vi "CommunicationTool.vi"(0 "VISA资源名称":refnum<visa-resource-name>="COM1", 1 "SN":string, 2 "ModelNumber":string, 5 "通信协议名称":string, 7 "Slot":T1, 9 "DelayTime":u32=1000, 11 "error in":errorcluster, 12 "Debug":bool) -> (3 "字符串数值":bool=TRUE, 4 "响应":string="ÿÿÿÿÿÿÿÿÿÿÿÿÿÿÿÿÿÿÿÿÿÿÿÿÿÿÿ", 6 "反馈结果":bool, 10 "CMD":string, 14 "data":string, 15 "error out":errorcluster)   [LabVIEW 2013]
doc: "本范例根据用户指示，对串口执行读写操作。范例运行时可按下“写入”或“读取”按钮，以及修改“读数”。\n\n设置的串口参数必须匹配连接仪器或设备的参数。本范例中，“读数”参数可指定串口读取的字节数。如端口字节超过指定的字节数，超出部分将不会被读取。如端口字节数少于指定的字节数，将返回超时错误。\n\n本范例可扩展流控制选项以包括XON和XOFF，从而允许用户选择控制字符。同时，用户可启用或禁用中止符。部分设备需要通过终止符确定命令字符串的结束位置。部分设备将发送终止符以说明待读取数据的末端。本范例演示了缓冲区中检测到终止符时，结束“读取”操作或添加终止符至“写入”数据末端的方法。"
uses:
  SystemCode/SysControl/Slot.ctl
  <vilib>/Utility/NIReport.llb/NI_report.lvclass
  SourceCode/PDINFO.ctl
  SourceCode/GlobalValue.vi
  <vilib>/Utility/error.llb/Error Cluster From Error Code.vi
  <vilib>/addons/_office/excel.llb/Excel Get Data ([str]).vi
  <vilib>/Utility/file.llb/Write To Spreadsheet File (string).vi
  <vilib>/Utility/file.llb/Read From Spreadsheet File (string).vi
  <vilib>/ErrorRing/Error Ring.xnode
  <vilib>/addons/_office/NI_ReportGenerationToolkit.lvlib
  <vilib>/Utility/NIReport.llb/Excel/NI_Excel.lvclass
panel:
  out "Time(ms)":u32
  out "SerNO":string
  out "硬件版本":string
  out "终端ID":string
  out "CCID":string="PASS"
  out "生产日期":string
  out "字符串":string
  out "x-y":u32
  out "已删除的部分":u8[](array[numeric]) format="%x"
  out "读取缓冲区":string
  out "数据Hex":string[](array[string])
  out "数据ASCII":string[](array[string])
  out "数据类型":string[](array[string])
  in  "命令列表":u16(ring)=17
  out "Write":bool
  out "Read":bool
  out "ConfigPath":string="C:\\Users\\dell\\Desktop\\ExcelReport.vi"
  out "Data":string
  out "DataType":string
  out "命令":string
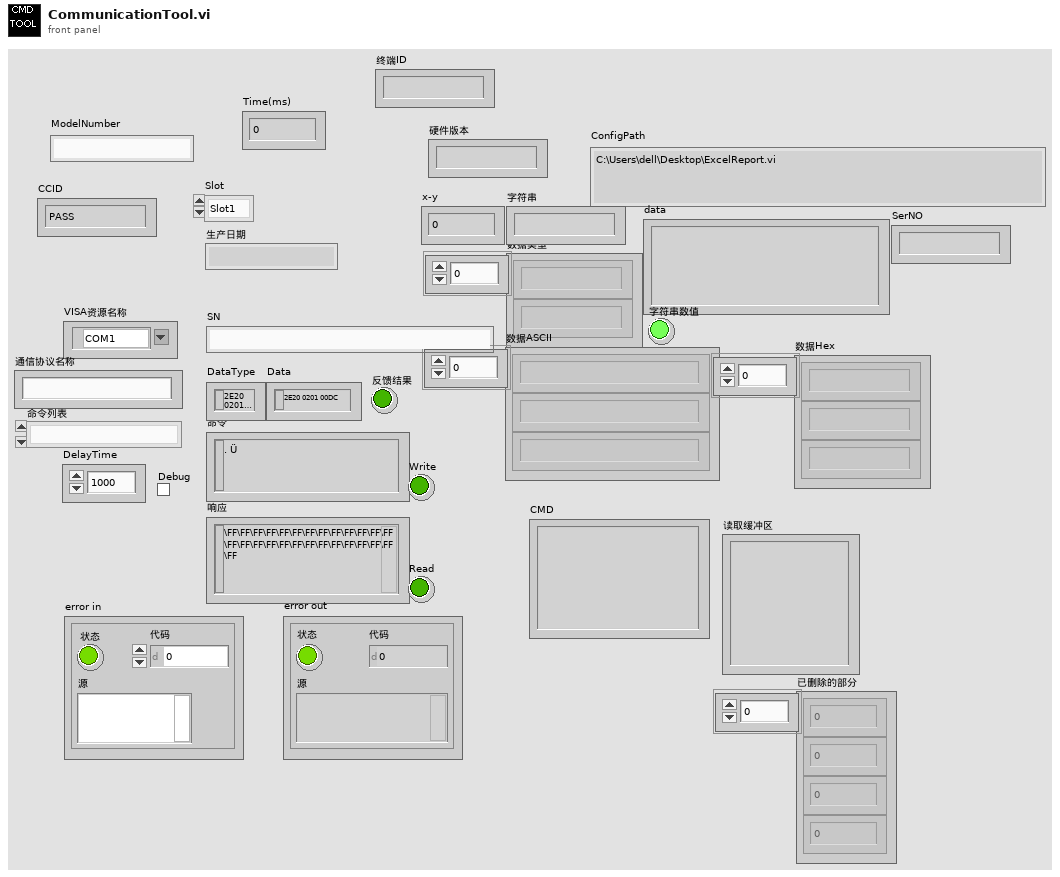
[diagram p1: front panel]
types:
  T1 = typedef "Slot.ctl" = enum16{"Slot1", "Slot2", "Slot3", "Slot4"}
  T2 = enum32{"invalid app kind", "Development System", "Run Time System", "Student Edition", "Embedded LabVIEW", "Evaluation", "Custom"}
  T3 = enum16{"maximized", "minimized", "normal", "no change"}
  T4 = enum16{"Standard Report", "HTML", "Word", "Excel"}
  T5 = typedef "PDINFO.ctl" = enum16{"Fw Ver", "HW Ver", "CCID", "WiFiName", "DevID", "SN", "TUID", "CertifID", "PdTime", "Provider", "WiFiPassword", "Imei", "AuthCode", "Reserved1", "Reserved2", "Reserved3"}
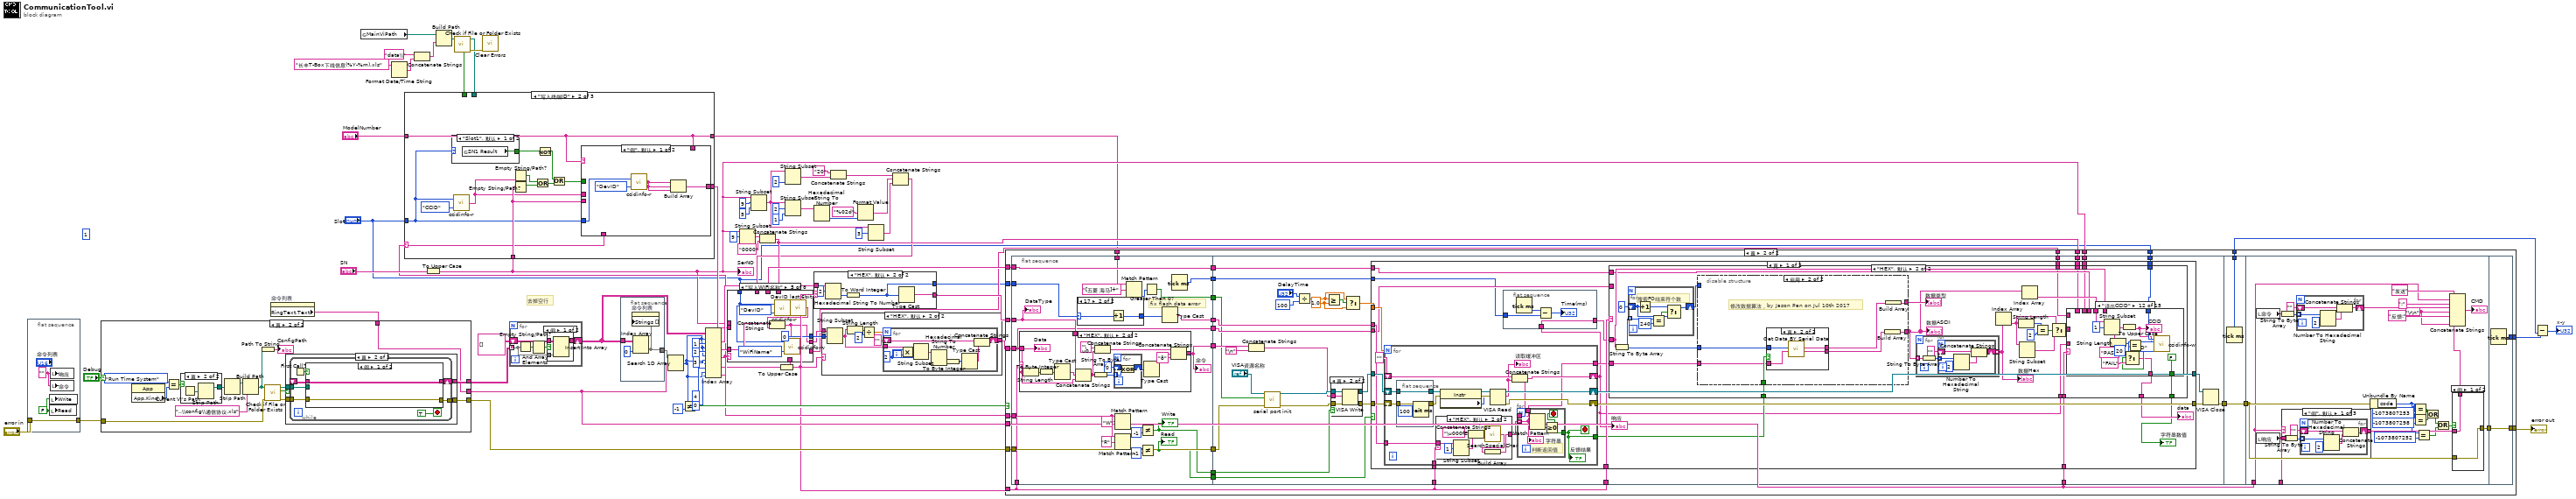
[diagram p0: block diagram]
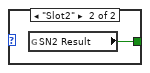
[diagram p3: hidden frame]
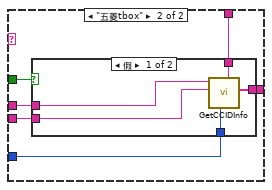
[diagram p4: hidden frame]
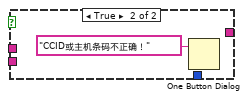
[diagram p5: hidden frame]
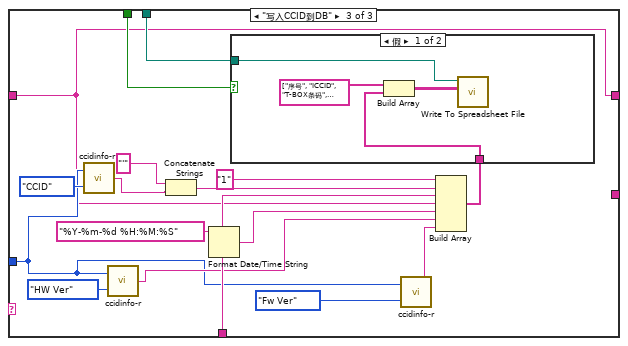
[diagram p6: hidden frame]
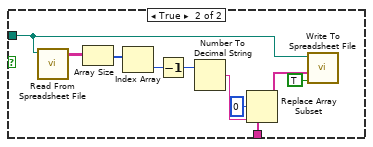
[diagram p7: hidden frame]
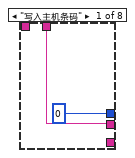
[diagram p8: hidden frame]
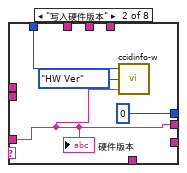
[diagram p9: hidden frame]
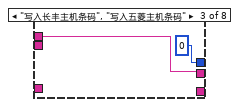
[diagram p10: hidden frame]
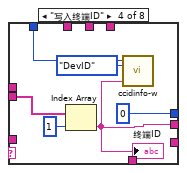
[diagram p11: hidden frame]
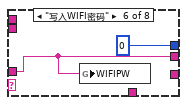
[diagram p12: hidden frame]
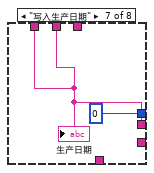
[diagram p13: hidden frame]
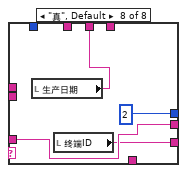
[diagram p14: hidden frame]
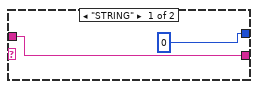
[diagram p15: hidden frame]
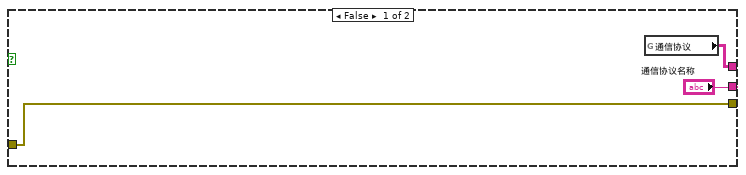
[diagram p18: hidden frame]
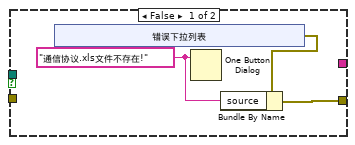
[diagram p19: hidden frame]
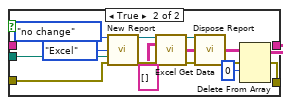
[diagram p20: hidden frame]
diagram:
  (unwired) 1
  # "去掉空行"
  n1 = flat-sequence {
    tunnel: "error in" -> [w71]
    tunnel: [w71] -> w68
    frame #0 {
      w73 = FALSE ("Read")
      w72 = "" ("响应")
      n2 = local write "Write"(w73) -> ()
      n3 = local write "Read"(w73) -> ()
      n4 = local write "响应"(w72) -> ()
      n5 = local write "命令"(w72) -> ()
    }
  }
  n6 = property on="命令列表" class="Ring (严格)"() -> ("RingText.Text"=w67:string)  [unwired: 2 in, 2 out]
  n7 = case shown="真" "Debug" {
    tunnel: [w75 w80] -> w65
    tunnel: w68 -> [w75 w79]
    tunnel: ["通信协议名称" w77] -> w56
    tunnel: [w74 w78] -> w5
    tunnel: w67 -> [_ w77]
    frame False {
      n8 = global read "GlobalValue.vi" "通信协议"() -> (w74:string[][])
    }
    frame True {
      n9 = property class="App"() -> ("App.Kind"=w89:T2)  [unwired: 2 in, 2 out]
      n10 = Equal?(x=T2."Run Time System" ("y"), y=w89) -> (x = y?=w91:bool)
      n11 = case shown="真" w91 {
        tunnel: [w125 w127] -> w90
        frame False {
          n12 = Current VI's Path() -> (path=w125:path)
        }
        frame True {
          n13 = Current VI's Path() -> (path=w126:path)
          n14 = Strip Path(path=w126) -> (stripped path=w127:path)  [unwired: 1 out]
        }
      }
      n15 = Strip Path(path=w90) -> (stripped path=w84:path)  [unwired: 1 out]
      n16 = Build Path(base path=w84, name or relative path="..\\config\\通信协议.xls" ("连接的字符串")) -> (appended path=w86:path)
      n17 = Path To String(path=w86) -> (string=→"ConfigPath":string)
      n18 = call <vilib>:"Check if File or Folder Exists.vi"("error in (no error)"=w79, "path"=w86) -> ("error out"=w81:errorcluster, "file or folder exists?"=w83:bool, "dup path"=w82:path)  [unwired: 7 out]
      n19 = case shown="真" w83 {
        tunnel: w82 -> [_ w102]
        tunnel: w81 -> [_ w101]
        tunnel: [w93 w100] -> w80
        tunnel: [_ w99] -> w78
        frame False {
          w94 = "通信协议.xls文件不存在!" ("消息")
          n20 = xnode "错误下拉列表"() -> ("错误输出"=w92:errorcluster)
          n21 = One Button Dialog(message=w94) -> ()  [unwired: 1 in, 1 out]
          n22 = Bundle By Name(cluster=w92, "source"=w94) -> (w93:errorcluster)
        }
        frame True {
          n23 = while {
            tunnel: w102 -> [w108]
            tunnel: [w107] -> w100
            tunnel: w101 -> [w106]
            shift-right: [w109] -> w99
            shift-left: _ -> [w104]
            stop <- TRUE stop-if-true
            n24 = First Call?() -> (First Call?: T/F=w103:bool)
            n25 = case shown="假" w103 {
              tunnel: [w111 w115] -> w109
              tunnel: w108 -> [_ w114]
              tunnel: [w110 w113] -> w107
              tunnel: w106 -> [w110 w112]
              tunnel: w104 -> [w111 _]
              frame False {
              }
              frame True {
                n26 = call <vilib>:"New Report.vi"("window state (normal)"=T3."no change", "report type"=T4."Excel", "template (empty)"=w114, "error in (no error)"=w112) -> ("report out"=w120:refnum<class "NI_report.lvclass">, "error out"=w121:errorcluster)  [unwired: 2 in, 8 out]
                n27 = call-poly <vilib>:"Excel Get Data.vi"("report in"=w120, "data type"=string[][] [], "error in (no error)"=w121) -> ("report out"=w117:refnum<class "NI_report.lvclass">, "data"=w122:string[][], "error out"=w116:errorcluster)  [unwired: 10 in]
                n28 = call-dynamic "Dispose Report.vi"("report in"=w117, "error in (no error)"=w116) -> ("error out"=w113:errorcluster)  [unwired: 3 in, 10 out]
                n29 = Delete From Array(array=w122, index (row)=0 ("索引 (行)")) -> (array with subset deleted=w115:string[][])  [unwired: 2 in, 1 out]
              }
            }
          }
        }
      }
    }
  }
  n30 = global read "GlobalValue.vi" "MainViPath"() -> (w11:path)
  n31 = Format Date/Time String(time format string (%c)="长丰T-Box下线信息(%Y-%m).xls" ("时间格式字符串(%c)")) -> (date/time string=w13:string)  [unwired: 2 in]
  n32 = Concatenate Strings("data\\" ("字符串"), w13) -> (w10:string)
  n33 = To Upper Case(1:"SN") -> (0:w15:string)
  "SerNO" <- w15
  n34 = Build Path(base path=w11, name or relative path=w10) -> (appended path=w9:path)
  n35 = call <vilib>:"Check if File or Folder Exists.vi"("path"=w9) -> ("error out"=w8:errorcluster, "file or folder exists?"=w6:bool, "dup path"=w7:path)  [unwired: 8 in]
  n36 = call <vilib>:"Clear Errors.vi"("error in (no error)"=w8) -> ()  [unwired: 6 in, 1 out]
  n37 = for {
    tunnel: w5 -> [w128] mode=indexing
    shift-right: [w131] -> w49
    shift-left: string[][] [] -> [w132]
    n38 = Empty String/Path?(string/path=w128) -> (empty?=w130:bool[])
    n39 = And Array Elements(Boolean array=w130) -> (logical AND=w129:bool)
    n40 = case shown="假" w129 {
      tunnel: w132 -> [w135 w136]
      tunnel: [w134 w136] -> w131
      tunnel: w128 -> [w133 _]
      frame False {
        n41 = Insert Into Array(array=w135, new element=w133) -> (w134:string[][])  [unwired: 2 in]
      }
      frame True {
      }
    }
  }
  n42 = flat-sequence {
    tunnel: [w138] -> w55
    tunnel: w49 -> [w137]
    frame #0 {
      n43 = Index Array(array=w137, index (col)=0 ("禁用的索引 (列)")) -> (element=w138:string[])  [unwired: 1 in]
      n44 = property on="命令列表" class="Ring (严格)"("Strings []"=w138) -> ()  [unwired: 2 in, 2 out]
    }
  }
  n45 = Search 1D Array(1D array=w55, element=w56) -> (index of element=w46:i32)  [unwired: 1 in]
  n46 = Not Equal?(x=w46, y=-1) -> (x != y?=w60:bool)
  n47 = Index Array(array=w49, index (row) #1=w46, index (col) #1=1 ("索引 (列)"), index (row) #2=w46, index (col) #2=2 ("索引 (列)"), index (row) #3=w46, index (col) #3=3 ("索引 (列)"), index (row) #4=w46, index (col) #4=4 ("禁用的索引 (列)"), index (row) #5=w46, index (col) #5=0 ("禁用的索引 (列)")) -> (element #1=w59:string, element #2=w44:string, element #3=w51:string, element #4=w53:string, element #5=w17:string)
  n48 = case shown="\"写入终端ID\"" w17 {
    selector: w17 -> [_ w143 _]
    tunnel: [_ w153 _] -> w20
    tunnel: "ModelNumber" -> [w140 w142 w172]
    tunnel: w15 -> [_ w146 w187]
    tunnel: w7 -> [_ _ w183]
    tunnel: w6 -> [_ _ w182]
    tunnel: "Slot" -> [_ w141 w174]
    tunnel: [w140 w142 w172] -> w2
    frame "假", Default {
    }
    frame "写入终端ID" {
      n49 = case shown="\"Slot1\", 默认" w141 {
        tunnel: [w154 w155] -> w152
        frame "Slot1", Default {
          n50 = global read "GlobalValue.vi" "SN1 Result"() -> (w154:bool)
        }
        frame "Slot2" {
          n51 = global read "GlobalValue.vi" "SN2 Result"() -> (w155:bool)
        }
      }
      n52 = call "ccidinfo-r.vi"("Data Type"=PDINFO."CCID", "Slot"=w141) -> ("Data"=w144:string)
      n53 = Empty String/Path?(string/path=w144) -> (empty?=w151:bool)
      n54 = Empty String/Path?(string/path=w146) -> (empty?=w150:bool)
      n55 = Or(x=w151, y=w150) -> (x .or. y?=w148:bool)
      n56 = Not(x=w152) -> (.not. x?=w149:bool)
      n57 = Or(x=w149, y=w148) -> (x .or. y?=w147:bool)
      n58 = case shown="\"假\", 默认" w142 {
        tunnel: [w159 w165] -> w153
        tunnel: w147 -> [_ w164]
        tunnel: w142 -> [_ w163]
        tunnel: w146 -> [_ w162]
        tunnel: w141 -> [w157 w161]
        tunnel: w144 -> [_ w160]
        tunnel: w143 -> [_ _]
        frame "假", Default {
          n59 = call "ccidinfo-r.vi"("Data Type"=PDINFO."DevID", "Slot"=w157) -> ("Data"=w156:string)
          n60 = Build Array(w156, w156, w156) -> (w159:string[])
        }
        frame "五菱tbox" {
          n61 = case shown="假" w164 {
            tunnel: [w170 _] -> w165
            tunnel: w160 -> [w169 _]
            tunnel: w162 -> [w168 _]
            tunnel: w163 -> [w167 _]
            tunnel: w161 -> [w166 _]
            frame False {
              n62 = call "GetCCIDInfo.vi"("table name"=w167, "Slot"=w166, "SerNO"=w168, "CCID"=w169) -> ("CCID信息"=w170:string[])  [unwired: 7 in]
            }
            frame True {
              n63 = One Button Dialog(message="CCID或主机条码不正确！" ("消息")) -> ()  [unwired: 1 in, 1 out]
            }
          }
        }
      }
    }
    frame "写入CCID到DB" {
      n64 = call "ccidinfo-r.vi"("Data Type"=PDINFO."CCID", "Slot"=w174) -> ("Data"=w178:string)
      n65 = call "ccidinfo-r.vi"("Data Type"=PDINFO."HW Ver", "Slot"=w174) -> ("Data"=w176:string)
      n66 = Concatenate Strings("'", w178) -> (w180:string)
      n67 = Format Date/Time String(time format string (%c)="%Y-%m-%d %H:%M:%S" ("时间格式字符串(%c)")) -> (date/time string=w185:string)  [unwired: 2 in]
      n68 = call "ccidinfo-r.vi"("Data Type"=PDINFO."Fw Ver", "Slot"=w174) -> ("Data"=w173:string)
      n69 = Build Array("1", w180, w187, w172, w185, w176, w173) -> (w184:string[])
      n70 = case shown="假" w182 {
        tunnel: w183 -> [w192 w193]
        tunnel: w184 -> [w191 w197]
        frame False {
          n71 = Build Array(string[] ["序号", "ICCID", "T-BOX条码", "设备型号", "生产日期", "硬件版本", "软件版本"], w191) -> (w190:string[][])
          n72 = call-poly <vilib>:"Write To Spreadsheet File.vi"("2D data"=w190, "file path (dialog if empty)"=w192) -> ()  [unwired: 6 in, 1 out]
        }
        frame True {
          n73 = call-poly <vilib>:"Read From Spreadsheet File.vi"("file path (dialog if empty)"=w193) -> ("all rows"=w202:string[][])  [unwired: 6 in, 4 out]
          n74 = Array Size(array=w202) -> (size(s)=w201:i32[])
          n75 = Index Array(array=w201) -> (element=w200:i32)  [unwired: 1 in]
          n76 = Decrement(x=w200) -> (x-1=w199:i32)
          n77 = Number To Decimal String(number=w199) -> (decimal integer string=w195:string)  [unwired: 1 in]
          n78 = Replace Array Subset(array=w197, new element=w195, index=0 ("索引")) -> (w194:string[])
          n79 = call-poly <vilib>:"Write To Spreadsheet File.vi"("append to file? (new file:F)"=TRUE, "1D data"=w194, "file path (dialog if empty)"=w193) -> ()  [unwired: 5 in, 1 out]
        }
      }
    }
  }
  n80 = String Subset(string=w15, offset (0)=9 ("偏移量(0)")) -> (substring=w39:string)  [unwired: 1 in]
  n81 = String Subset(string=w15, offset (0)=9 ("偏移量(0)"), length (rest)=5 ("长度（剩余）")) -> (substring=w27:string)
  n82 = Concatenate Strings(w39, "0000" ("字符串")) -> (w37:string)
  n83 = To Upper Case(1:w51) -> (0:w3:string)
  n84 = String Subset(string=w27, length (rest)=2 ("长度（剩余）")) -> (substring=w34:string)  [unwired: 1 in]
  n85 = String Subset(string=w27, offset (0)=2 ("偏移量(0)"), length (rest)=1 ("长度（剩余）")) -> (substring=w29:string)
  n86 = Hexadecimal String To Number(string=w29) -> (number=w24:u32)  [unwired: 2 in, 1 out]
  n87 = case shown="\"HEX\", 默认" w3 {
    tunnel: w59 -> [w204 w207]
    tunnel: [w204 w206] -> w58
    tunnel: [i16 0 w205] -> w1
    frame "STRING" {
    }
    frame "HEX", Default {
      n88 = Hexadecimal String To Number(string=w207, offset=2 ("偏移量")) -> (number=w209:u32)  [unwired: 1 in, 1 out]
      n89 = To Word Integer(number=w209) -> (16bit integer=w205:i16)
      n90 = Type Cast(x=w205) -> (*(type *) &x=w206:string)  [unwired: 1 in]
    }
  }
  n91 = Concatenate Strings("20" ("字符串"), w34) -> (w26:string)
  n92 = Format Value(format string="%02d" ("格式字符串"), value (0)=w24) -> (output string=w22:string)  [unwired: 1 in]
  n93 = String Subset(string=w27, offset (0)=3 ("偏移量(0)")) -> (substring=w25:string)  [unwired: 1 in]
  n94 = Concatenate Strings(w26, w22, w25) -> (w21:string)
  n95 = case shown="\"写入WIFI名称\"" w17 {
    tunnel: w44 -> [_ w212 _ _ w230 w232 _ w239]
    tunnel: [w210 w212 w216 w218 w226 w232 w234 w239] -> w19
    tunnel: [0 ("偏移量(0)") 0 ("偏移量(0)") 0 ("偏移量(0)") 0 ("偏移量(0)") 0 ("偏移量(0)") 0 ("偏移量(0)") 0 ("偏移量(0)") 2 ("偏移量(0)")] -> w43
    tunnel: [_ _ _ _ _ _ w234 w237] -> w41
    tunnel: w37 -> [w210 _ _ _ _ _ _ _]
    tunnel: w21 -> [_ _ _ _ _ _ w234 _]
    tunnel: w15 -> [_ _ w216 _ _ _ _ _]
    tunnel: w20 -> [_ _ _ w222 _ _ _ _]
    tunnel: [_ _ _ _ _ _ _ w236] -> w18
    tunnel: "Slot" -> [_ w214 _ w219 w227 _ _ _]
    tunnel: w3 -> [_ _ _ _ _ _ _ _]
    frame "写入主机条码" {
    }
    frame "写入硬件版本" {
      n96 = call "ccidinfo-w.vi"("Data"=w212, "Data Type"=PDINFO."HW Ver", "Slot"=w214) -> ()  [unwired: 1 in]
      "硬件版本" <- w212
    }
    frame "写入长丰主机条码", "写入五菱主机条码" {
    }
    frame "写入终端ID" {
      n97 = Index Array(array=w222, index=1 ("索引")) -> (element=w218:string)
      "终端ID" <- w218
      n98 = call "ccidinfo-w.vi"("Data"=w218, "Data Type"=PDINFO."DevID", "Slot"=w219) -> ()  [unwired: 1 in]
    }
    frame "写入WIFI名称" {
      n99 = call "ccidinfo-r.vi"("Data Type"=PDINFO."DevID", "Slot"=w227) -> ("Data"=w225:string)
      n100 = call "DevID last 6bit.vi"("Devid"=w225) -> ("结果字符串"=w224:string)  [unwired: 4 in]
      n101 = Concatenate Strings(w230, w224) -> (w226:string)
      n102 = call "ccidinfo-w.vi"("Data"=w226, "Data Type"=PDINFO."WiFiName", "Slot"=w227) -> ()  [unwired: 1 in]
    }
    frame "写入WIFI密码" {
      n103 = global write "GlobalValue.vi" "WIFIPW"(w232) -> ()
    }
    frame "写入生产日期" {
      "生产日期" <- w234
    }
    frame "真", Default {
      n104 = local read "生产日期"() -> (w237:string)
      n105 = local read "终端ID"() -> (w236:string)
    }
  }
  n106 = case shown="\"HEX\", 默认" w3 {
    tunnel: [w240 w245] -> w57
    tunnel: w19 -> [w240 w244]
    tunnel: w43 -> [_ w241]
    frame "ASCII" {
    }
    frame "HEX", Default {
      n107 = String Subset(string=w244, offset (0)=w241) -> (substring=w243:string)  [unwired: 1 in]
      n108 = String Length(string=w243) -> (length=w247:i32)
      n109 = Divide(x=w247, y=2) -> (x/y=w242:dbl)
      n110 = for {
        N: w242 -> [_]
        tunnel: w243 -> [w253]
        shift-right: [w255] -> w245
        shift-left: "" -> [w254]
        i -> [w251]
        w249 = 2 ("x")
        n111 = Multiply(x=w249, y=w251) -> (x*y=w250:i32)
        n112 = String Subset(string=w253, offset (0)=w250, length (rest)=w249) -> (substring=w252:string)
        n113 = Hexadecimal String To Number(string=w252) -> (number=w258:u32)  [unwired: 2 in, 1 out]
        n114 = To Byte Integer(number=w258) -> (8bit integer=w257:i8)
        n115 = Type Cast(x=w257) -> (*(type *) &x=w256:string)  [unwired: 1 in]
        n116 = Concatenate Strings(w254, w256) -> (w255:string)
      }
    }
  }
  n117 = case shown="真" w60 {
    tunnel: w56 -> [w263 w280]
    tunnel: w58 -> [_ w291]
    tunnel: w57 -> [_ w290]
    tunnel: w65 -> [_ w289]
    tunnel: [w259 w287] -> w70
    tunnel: w53 -> [_ w286]
    tunnel: w3 -> [_ w281]
    tunnel: [_ w276] -> w66
    tunnel: [_ w275] -> w48
    tunnel: w41 -> [_ w274]
    tunnel: w37 -> [_ w272]
    tunnel: w15 -> [_ w271]
    tunnel: w18 -> [_ w270]
    tunnel: "Slot" -> [_ w267]
    tunnel: w2 -> [_ w266]
    tunnel: w1 -> [_ w264]
    frame False {
      (unwired) "FF" ("响应")
      n118 = Concatenate Strings(w263, "名称不存在" ("消息")) -> (w260:string)
      n119 = One Button Dialog(message=w260) -> ()  [unwired: 1 in, 1 out]
      n120 = Bundle By Name(cluster=errorcluster {"status"=TRUE, "code"=5000, "source"=""} ("error in 1 (no error)"), "source"=w260) -> (w259:errorcluster)
    }
    frame True {
      n121 = flat-sequence {
        tunnel: w291 -> [w303]
        tunnel: w290 -> [w300]
        tunnel: w289 -> [w314]
        tunnel: [w314] -> w288
        tunnel: w286 -> [w313]
        tunnel: [w306] -> w285
        tunnel: [w305] -> w284
        tunnel: [w304] -> w283
        tunnel: [w292] -> w282
        tunnel: w281 -> [w302]
        tunnel: w274 -> [w301]
        tunnel: [w301] -> w273
        tunnel: [w300] -> w269
        tunnel: [w299] -> w268
        tunnel: w266 -> [w298]
        tunnel: [w295] -> w265
        tunnel: w264 -> [w294]
        tunnel: w288 -> [w367]
        tunnel: w285 -> [w362]
        tunnel: w284 -> [w365]
        tunnel: [w366] -> w279
        tunnel: w283 -> [w341]
        tunnel: w282 -> [w361]
        tunnel: w281 -> [w352]
        tunnel: w281 -> [w351]
        tunnel: w280 -> [w350]
        tunnel: w273 -> [w349]
        tunnel: w272 -> [w348]
        tunnel: w271 -> [w347]
        tunnel: w270 -> [w346]
        tunnel: w269 -> [w345]
        tunnel: w268 -> [w344]
        tunnel: w267 -> [w343]
        tunnel: w265 -> [w338]
        tunnel: w279 -> [w716]
        tunnel: [w716] -> w278
        tunnel: [w715] -> w275
        tunnel: w278 -> [w729]
        tunnel: w280 -> [w717]
        tunnel: [w718] -> _
        tunnel: [w730] -> w277
        tunnel: [w762] -> w287
        tunnel: w277 -> [w762]
        tunnel: [w761] -> w276
        frame #0 {
          # "fix flash data error"
          n122 = case shown="\"HEX\", 默认" w302 {
            tunnel: w300 -> [w319 w331]
            tunnel: [w318 w325] -> w304
            tunnel: w303 -> [w320 w324]
            frame "STRING" {
              n123 = Concatenate Strings(w320, w319) -> (w318:string)
            }
            frame "HEX", Default {
              n124 = String Length(string=w331) -> (length=w322:i32)
              n125 = To Byte Integer(number=w322) -> (8bit integer=w323:i8)
              n126 = Type Cast(x=w323) -> (*(type *) &x=w321:string)  [unwired: 1 in]
              n127 = Concatenate Strings(w324, w321, w331) -> (w334:string)
              n128 = String To Byte Array(string=w334) -> (unsigned byte array=w330:u8[])
              n129 = Concatenate Strings("\u000f" ("HeadCode"), w334) -> (w327:string)
              n130 = for {
                tunnel: w330 -> [w337] mode=indexing
                shift-right: [w335] -> w328
                shift-left: u8 0 ("y") -> [w336]
                n131 = Exclusive Or(1:w337, 2:w336) -> (0:w335:u8)
              }
              n132 = Type Cast(x=w328) -> (*(type *) &x=w332:string)  [unwired: 1 in]
              n133 = Concatenate Strings(w327, w332, "ð" ("字符串")) -> (w325:string)
              "Data" <- w331
            }
          }
          "命令" <- w304
          n134 = case shown="17" w294 {
            selector: w294 -> [w315 w317]
            tunnel: [w315 w316] -> w293
            frame 0, Default {
            }
            frame 17 {
              n135 = Increment(x=w317) -> (x+1=w316:i16)
            }
          }
          n136 = Match Pattern(string=w313, regular expression="W" ("正则表达式")) -> (offset past match=w307:i32)  [unwired: 1 in, 3 out]
          n137 = Match Pattern(string=w313, regular expression="R" ("正则表达式")) -> (offset past match=w308:i32)  [unwired: 1 in, 3 out]
          n138 = Match Pattern(string=w298, regular expression="[五菱 海马]+" ("正则表达式")) -> (offset past match=w296:i32)  [unwired: 1 in, 3 out]
          n139 = Not Equal?(x=w307, y=-1) -> (x != y?=w306:bool)
          "Write" <- w306
          n140 = Not Equal?(x=w308, y=-1) -> (x != y?=w305:bool)
          "Read" <- w305
          n141 = Greater Than 0?(x=w296) -> (x > 0?=w295:bool)
          n142 = Type Cast(x=w293) -> (*(type *) &x=w292:string)  [unwired: 1 in]
          n143 = Tick Count (ms)() -> (millisecond timer value=w299:u32)
          "DataType" <- w303
        }
        frame #1 {
          w358 = 1.0 ("y")
          n144 = Concatenate Strings(w341, "\n") -> (w339:string)
          n145 = call "serial port init.vi"("错误输入（无错误）"=w367, "海马(1)"=w338, "VISA引用句柄输入"="VISA资源名称") -> ("错误输出"=w363:errorcluster, "VISA引用句柄输出"=w364:refnum<visa-resource-name>)  [unwired: 7 in]
          n146 = Divide(x="DelayTime", y=u32 100) -> (x/y=w357:dbl)
          n147 = Greater Or Equal?(x=w357, y=w358) -> (x >= y?=w356:bool)
          n148 = case shown="真" w362 {
            tunnel: w364 -> [w371 w376]
            tunnel: [w371 w375] -> w360
            tunnel: [w370 w374] -> w359
            tunnel: w363 -> [w370 w373]
            tunnel: w339 -> [_ w372]
            frame False {
            }
            frame True {
              n149 = VISA Write(VISA resource name=w376, write buffer=w372, error in (no error)=w373) -> (VISA resource name out=w375:refnum<visa-resource-name>, error out=w374:errorcluster)  [unwired: 1 out]
            }
          }
          n150 = Select(t=w357, s=w356, f=w358) -> (s? t:f=w353:dbl)
          n151 = case shown="真" w365 {
            tunnel: [w398 w714] -> w368
            tunnel: w360 -> [w397 w714]
            tunnel: [w399 w713] -> w369
            tunnel: w359 -> [w396 w713]
            tunnel: w361 -> [w394 _]
            tunnel: w353 -> [w393 _]
            tunnel: w352 -> [w392 _]
            tunnel: w351 -> [w391 _]
            tunnel: w350 -> [w389 _]
            tunnel: w349 -> [w386 _]
            tunnel: w348 -> [w385 _]
            tunnel: w347 -> [w384 _]
            tunnel: w346 -> [w383 _]
            tunnel: w345 -> [w382 _]
            tunnel: w344 -> [w381 _]
            tunnel: w343 -> [w379 _]
            frame True {
              n152 = for {
                N: w393 -> [_]
                shift-right: [w697] -> w399
                shift-left: w396 -> [w687]
                shift-right: [w685] -> w377
                shift-left: "" ("read buffer") -> [w692]
                shift-right: [w696] -> w398
                shift-left: w397 -> [w686]
                tunnel: w394 -> [w682]
                tunnel: w392 -> [w684]
                tunnel: [w683] -> w390
                tunnel: [w681] -> w378
                stop <- w683 stop-if-true
                n153 = flat-sequence {
                  tunnel: w687 -> [w712]
                  tunnel: [w712] -> w688
                  tunnel: [w711] -> w689
                  tunnel: w686 -> [w711]
                  frame #0 {
                    n154 = Wait (ms)(milliseconds to wait=u32 100 ("等待时间（毫秒）")) -> ()  [unwired: 1 out]
                  }
                }
                n155 = case shown="\"HEX\", 默认" w684 {
                  tunnel: [string[] ["0x0000000", "create auto test task"] w703] -> w691
                  tunnel: w682 -> [_ w709]
                  frame "STRING" {
                  }
                  frame "HEX", Default {
                    n156 = String Subset(string=w709, offset (0)=1 ("偏移量(0)")) -> (substring=w706:string)  [unwired: 1 in]
                    n157 = Concatenate Strings("\u000f€" ("正则表达式"), w706) -> (w705:string)
                    n158 = call "SearchSpecialChar.vi"("正则表达式"=w705) -> ("字符串"=w704:string)
                    n159 = Build Array(w704) -> (w703:string[])
                  }
                }
                n160 = property class="Instr"(reference=w689, error in=w688) -> (reference out=w695:refnum<visa-resource-name>, error out=w694:errorcluster, "Serial Settings:Number of Bytes at Serial Port"=w693:u32)
                n161 = VISA Read(VISA resource name=w695, byte count=w693, error in (no error)=w694) -> (VISA resource name out=w696:refnum<visa-resource-name>, read buffer=w690:string, error out=w697:errorcluster)  [unwired: 1 out]
                "读取缓冲区" <- w690
                n162 = Concatenate Strings(w692, w690) -> (w685:string)
                n163 = for {
                  tunnel: w691 -> [w698] mode=indexing
                  tunnel: w685 -> [w700]
                  tunnel: [w699] -> w683
                  tunnel: [w698] -> w681
                  stop <- w699 stop-if-true
                  # "判断返回值"
                  n164 = Match Pattern(string=w700, regular expression=w698) -> (offset past match=w701:i32)  [unwired: 1 in, 3 out]
                  n165 = Greater Or Equal To 0?(x=w701) -> (x >= 0?=w699:bool)
                  "字符串" <- w698
                }
                "反馈结果" <- w683
              }
              "响应" <- w377
              n166 = flat-sequence {
                tunnel: w381 -> [w401]
                tunnel: w377 -> [w400]
                tunnel: [w400] -> w380
                frame #0 {
                  n167 = Tick Count (ms)() -> (millisecond timer value=w402:u32)
                  n168 = Subtract(x=w402, y=w401) -> (x-y=→"Time(ms)":u32)
                }
              }
              n169 = case shown="\"HEX\", 默认" w391 {
                tunnel: w380 -> [w410 w481]
                tunnel: w390 -> [w407 w473]
                tunnel: w389 -> [w411 w489]
                tunnel: [w409 w488] -> w388
                tunnel: [w408 w487] -> w387
                tunnel: w386 -> [_ w478]
                tunnel: w385 -> [_ w477]
                tunnel: w384 -> [w405 w476]
                tunnel: w383 -> [_ w475]
                tunnel: w382 -> [w406 _]
                tunnel: w379 -> [w404 w474]
                tunnel: w378 -> [_ w472]
                tunnel: w377 -> [_ w471]
                frame "STRING" {
                  n170 = case shown="\"查询版本(1701)\"" w411 {
                    tunnel: [w412 w421 w444] -> w409
                    tunnel: [FALSE FALSE FALSE] -> w408
                    tunnel: w410 -> [_ w428 w452]
                    tunnel: w407 -> [w413 _ _]
                    tunnel: w406 -> [_ w423 w446]
                    tunnel: w405 -> [_ _ _]
                    tunnel: w404 -> [_ w419 w442]
                    frame "真", Default {
                      n171 = Select(t="OK", s=w413, f="") -> (s? t:f=w412:string)
                    }
                    frame "查询版本", "查询版本(长丰)" {
                      # "查询版本指令--修改兼容海马,五菱,长丰  --- by Jason Pan on Jan 20th 2017"
                      n172 = Concatenate Strings(w423, "\n" ("字符串")) -> (w422:string)
                      n173 = Match Pattern(string=w428, regular expression=w422) -> (after substring=w427:string)  [unwired: 1 in, 3 out]
                      n174 = for {
                        tunnel: w427 -> [w441]
                        tunnel: [w440] -> w425
                        tunnel: string[] ["\r\n\t1, 0x00000001\r\ncmd>", "\r\n\t0, 0x00000000\r\ncmd>", "\n\t0, 0x00000000", "\r\ncmd>"] -> [w437] mode=indexing
                        tunnel: [w436] -> w426
                        i -> [w436]
                        stop <- w438 stop-if-true
                        n175 = Match Pattern(string=w441, regular expression=w437) -> (before substring=w440:string, offset past match=w439:i32)  [unwired: 1 in, 2 out]
                        n176 = Greater Or Equal To 0?(x=w439) -> (x >= 0?=w438:bool)
                      }
                      n177 = case shown="0, 默认" w426 {
                        tunnel: [w430 w431] -> w424
                        tunnel: w425 -> [w430 w435]
                        frame 0, Default {
                          # "海马/长丰tbox"
                        }
                        frame 3 {
                          # "五菱tbox"
                          n178 = Match Pattern(string=w435, regular expression="app start,version:" ("正则表达式")) -> (after substring=w433:string)  [unwired: 1 in, 3 out]
                          n179 = Match Pattern(string=w433, regular expression="\r\n" ("正则表达式")) -> (before substring=w431:string)  [unwired: 1 in, 3 out]
                        }
                      }
                      n180 = call <vilib>:"Trim Whitespace.vi"("string"=w424) -> ("trimmed string"=w421:string)  [unwired: 1 in]
                      n181 = call "ccidinfo-w.vi"("Data"=w421, "Data Type"=PDINFO."Fw Ver", "Slot"=w419) -> ()  [unwired: 1 in]
                    }
                    frame "查询版本(1701)" {
                      # "查询版本指令--修改兼容海马,五菱,长丰  --- by Jason Pan on Jan 20th 2017"
                      n182 = Concatenate Strings(w446) -> (w445:string)
                      n183 = Match Pattern(string=w452, regular expression=w445) -> (after substring=w451:string)  [unwired: 1 in, 3 out]
                      n184 = for {
                        tunnel: w451 -> [w470]
                        tunnel: [w469] -> w448
                        tunnel: string[] ["\r\nAES", "\nAES"] -> [w466] mode=indexing
                        tunnel: [w465] -> w449
                        i -> [w465]
                        stop <- w467 stop-if-true
                        n185 = Match Pattern(string=w470, regular expression=w466) -> (before substring=w469:string, offset past match=w468:i32)  [unwired: 1 in, 2 out]
                        n186 = Greater Or Equal To 0?(x=w468) -> (x >= 0?=w467:bool)
                      }
                      n187 = case shown="0" w449 {
                        tunnel: [w454 w455 w460] -> w447
                        tunnel: w448 -> [w454 w459 w464]
                        frame -1, Default {
                          # "海马/长丰tbox"
                        }
                        frame 0 {
                          # "tbox/1701"
                          n188 = Match Pattern(string=w459, regular expression="app start,version:" ("正则表达式")) -> (after substring=w457:string)  [unwired: 1 in, 3 out]
                          n189 = Match Pattern(string=w457, regular expression="\r\n" ("正则表达式")) -> (before substring=w455:string)  [unwired: 1 in, 3 out]
                        }
                        frame 1 {
                          # "1701"
                          n190 = Match Pattern(string=w464, regular expression="app start,version:" ("正则表达式")) -> (after substring=w462:string)  [unwired: 1 in, 3 out]
                          n191 = Match Pattern(string=w462, regular expression="\n" ("正则表达式")) -> (before substring=w460:string)  [unwired: 1 in, 3 out]
                        }
                      }
                      n192 = call <vilib>:"Trim Whitespace.vi"("string"=w447) -> ("trimmed string"=w444:string)  [unwired: 1 in]
                      n193 = call "ccidinfo-w.vi"("Data"=w444, "Data Type"=PDINFO."Fw Ver", "Slot"=w442) -> ()  [unwired: 1 in]
                    }
                  }
                }
                frame "HEX", Default {
                  n194 = String To Byte Array(string=w481) -> (unsigned byte array=w486:u8[])
                  n195 = for {
                    tunnel: w486 -> [w555] mode=indexing
                    shift-right: [w551] -> w484
                    shift-left: 0 ("y") -> [w550]
                    # "搜索FO结束符个数"
                    n196 = Increment(x=w550) -> (x+1=w552:i32)
                    n197 = Equal?(x=w555, y=u8 240) -> (x = y?=w553:bool)
                    n198 = Select(t=w552, s=w553, f=w550) -> (s? t:f=w551:i32)
                  }
                  n199 = disable-structure shown="启用" {
                    disable-tunnel: w486 -> [w499 w535]
                    disable-tunnel: w484 -> [w498 _]
                    disable-tunnel: [w497 w533] -> w483
                    disable-tunnel: [w496 w532] -> w480
                    disable-tunnel: w473 -> [_ w530]
                    disable-tunnel: w472 -> [_ w529]
                    frame Disabled {
                      n200 = for {
                        N: w498 -> [_]
                        shift-right: [w522] -> _
                        shift-left: w499 -> [w523]
                        tunnel: [w506] -> w496 mode=indexing
                        tunnel: [w502] -> w497 mode=indexing
                        stop <- w520 stop-if-true
                        # "删除数据类型和两位长度，删除校验码"
                        # "下一个OF和FO的消息处理"
                        # "获取OF和FO之间的数据"
                        n201 = Search 1D Array(1D array=w523, element=u8 15 ("元素")) -> (index of element=w525:i32)  [unwired: 1 in]
                        n202 = Search 1D Array(1D array=w523, element=u8 240 ("元素")) -> (index of element=w518:i32)  [unwired: 1 in]
                        n203 = Increment(x=w525) -> (x+1=w524:i32)
                        n204 = Equal?(x=w518, y=-1) -> (x = y?=w520:bool)
                        n205 = Subtract(x=w518, y=w524) -> (x-y=w526:i32)
                        n206 = Increment(x=w518) -> (x+1=w519:i32)
                        n207 = Array Subset(array=w523, index=w524, length=w526) -> (w515:u8[])
                        n208 = Array Subset(array=w523, index=w519) -> (w522:u8[])  [unwired: 1 in]
                        n209 = Index Array(array=w515) -> (element #1=w516:u8, element #2=w505:u8)  [unwired: 2 in]
                        n210 = Delete From Array(array=w515, length=3 ("长度"), index=0 ("索引")) -> (deleted portion=→"已删除的部分":u8[], array with subset deleted=w512:u8[])
                        n211 = Reverse 1D Array(array=w512) -> (reversed array=w511:u8[])
                        n212 = Number To Hexadecimal String(1:i16 2 ("宽度(-)"), 2:w516) -> (0:w503:string)
                        n213 = Number To Hexadecimal String(1:i16 2 ("宽度(-)"), 2:w505) -> (0:w504:string)
                        n214 = Delete From Array(array=w511, length=1 ("长度"), index=0 ("索引")) -> (array with subset deleted=w508:u8[])  [unwired: 1 out]
                        n215 = Reverse 1D Array(array=w508) -> (reversed array=w507:u8[])
                        n216 = Concatenate Strings(w503, w504) -> (w502:string)
                        n217 = Byte Array To String(unsigned byte array=w507) -> (string=w506:string)
                      }
                    }
                    frame Enabled {
                      # "修改数据算法，by Jason Pan on Jul 10th 2017"
                      n218 = case shown="真" w530 {
                        tunnel: w535 -> [_ w540]
                        tunnel: [w536 w539] -> w534
                        tunnel: [w536 w538] -> w531
                        tunnel: w529 -> [_ w537]
                        frame False {
                          w536 = ""
                        }
                        frame True {
                          n219 = call "Get Data BY Serial Data.vi"("HEAD"=w537, "Data in"=w540) -> ("Data"=w538:string, "Data Type"=w539:string)  [unwired: 8 in]
                        }
                      }
                      n220 = Build Array(w531) -> (w532:string[])
                      n221 = Build Array(w534) -> (w533:string[])
                    }
                  }
                  "数据类型" <- w483
                  "数据ASCII" <- w480
                  n222 = for {
                    tunnel: w480 -> [w544] mode=indexing
                    tunnel: [w541] -> w482 mode=indexing
                    n223 = String To Byte Array(string=w544) -> (unsigned byte array=w542:u8[])
                    n224 = for {
                      tunnel: w542 -> [w549] mode=indexing
                      shift-right: [w547] -> w541
                      shift-left: "" -> [w546]
                      n225 = Number To Hexadecimal String(1:i16 2 ("宽度(-)"), 2:w549) -> (0:w548:string)
                      n226 = Concatenate Strings(w546, w548) -> (w547:string)
                    }
                  }
                  "数据Hex" <- w482
                  n227 = Index Array(array=w482) -> (element=w492:string)  [unwired: 1 in]
                  n228 = String Length(string=w492) -> (length=w495:i32)
                  n229 = String Subset(string=w492) -> (substring=w491:string)  [unwired: 2 in]
                  n230 = Index Array(array=w480) -> (element=w479:string)  [unwired: 1 in]
                  n231 = Equal?(x=w495, y=2) -> (x = y?=w493:bool)
                  n232 = Select(t=w492, s=w493, f=w491) -> (s? t:f=w490:string)
                  n233 = case shown="\"读出CCID\"" w489 {
                    tunnel: w490 -> [w558 w571 w575 w578 w589 _ _ _ _ _ _ _ _ _ _]
                    tunnel: [w557 w567 w573 w579 w586 w595 w598 w606 w619 w627 w637 w645 w656 w666 w676] -> w488
                    tunnel: [TRUE TRUE TRUE FALSE FALSE FALSE TRUE FALSE FALSE FALSE FALSE FALSE FALSE FALSE FALSE] -> w487
                    tunnel: w481 -> [_ _ _ _ _ _ w602 _ _ _ _ _ _ _ _]
                    tunnel: w479 -> [_ _ _ _ _ _ _ w610 w618 w625 w634 w653 w660 w663 w674]
                    tunnel: w478 -> [_ _ _ _ _ _ _ _ _ _ _ _ w655 _ _]
                    tunnel: w477 -> [_ _ _ _ _ _ _ w604 _ _ _ _ _ _ _]
                    tunnel: w476 -> [_ _ _ _ _ _ _ _ _ _ w635 _ _ _ _]
                    tunnel: w475 -> [_ _ _ _ _ _ _ _ _ _ _ _ _ w665 _]
                    tunnel: w474 -> [_ _ _ _ _ _ _ _ w613 _ _ w644 _ _ w672]
                    tunnel: w471 -> [_ _ _ _ _ w596 _ _ _ _ _ _ _ _ _]
                    frame "查询BAT7.2V_DET电压" {
                      n234 = Hexadecimal String To Number(string=w558) -> (number=w561:u32)  [unwired: 2 in, 1 out]
                      n235 = Divide(x=w561, y=u32 1000) -> (x/y=w559:dbl)
                      n236 = Number To Fractional String(number=w559) -> (F-format string=w557:string)  [unwired: 3 in]
                    }
                    frame "查询BAT_DET状态" {
                      n237 = Hexadecimal String To Number(string=w571) -> (number=w569:u32)  [unwired: 2 in, 1 out]
                      n238 = Multiply(x=w569, y=u32 11) -> (x*y=w568:u32)
                      n239 = Divide(x=w568, y=u32 1000) -> (x/y=w564:dbl)
                      n240 = Add(x=w564, y=0.3) -> (x+y=w562:dbl)
                      n241 = Number To Fractional String(number=w562) -> (F-format string=w567:string)  [unwired: 3 in]
                    }
                    frame "加速度传感器返回数据1" {
                      n242 = Hexadecimal String To Number(string=w575) -> (number=w574:u32)  [unwired: 2 in, 1 out]
                      n243 = Number To Decimal String(number=w574) -> (decimal integer string=w573:string)  [unwired: 1 in]
                    }
                    frame "真", Default {
                      n244 = Empty String/Path?(string/path=w578) -> (empty?=w577:bool)
                      n245 = case shown="假" w577 {
                        tunnel: [w581 ""] -> w579
                        tunnel: w578 -> [w580 _]
                        frame False {
                          n246 = Concatenate Strings("0x" ("字符串"), w580) -> (w581:string)
                        }
                        frame True {
                        }
                      }
                    }
                    frame "查询平台登录状态" {
                      n247 = Empty String/Path?(string/path=w589) -> (empty?=w588:bool)
                      n248 = case shown="假" w588 {
                        tunnel: [w592 ""] -> w590
                        tunnel: w589 -> [w591 _]
                        frame False {
                          n249 = Concatenate Strings("0x" ("字符串"), w591) -> (w592:string)
                        }
                        frame True {
                        }
                      }
                      n250 = String Subset(string=w590, offset (0)=0 ("长度（剩余）"), length (rest)=4 ("长度（剩余）")) -> (substring=w586:string)
                    }
                    frame "查询4G固件版本" {
                      n251 = call "VerStringTrim.vi"("读取缓冲区"=w596) -> ("结果"=w595:string)
                    }
                    frame "查询版本" {
                      n252 = Match Pattern(string=w602, regular expression="ver()\r\n" ("正则表达式")) -> (after substring=w600:string)  [unwired: 1 in, 3 out]
                      n253 = Match Pattern(string=w600, regular expression="\r\n\t1, 0x00000001\r\ncmd>" ("正则表达式")) -> (before substring=w598:string)  [unwired: 1 in, 3 out]
                    }
                    frame "读出主机条码" {
                      n254 = To Upper Case(1:w604) -> (0:w605:string)
                      n255 = Equal?(x=w610, y=w605) -> (x = y?=w609:bool)
                      n256 = Select(t="PASS" ("string"), s=w609, f="FAIL") -> (s? t:f=w606:string)
                    }
                    frame "读出WIFI名称" {
                      n257 = call "ccidinfo-r.vi"("Data Type"=PDINFO."WiFiName", "Slot"=w613) -> ("Data"=w612:string)
                      n258 = To Upper Case(1:w612) -> (0:w616:string)
                      n259 = Match Pattern(string=w618, regular expression=w616) -> (match substring=w617:string)  [unwired: 1 in, 3 out]
                      n260 = Equal?(x=w617, y=w616) -> (x = y?=w615:bool)
                      n261 = Select(t="PASS" ("string"), s=w615, f="FAIL") -> (s? t:f=w619:string)
                    }
                    frame "读出WIFI密码" {
                      n262 = global read "GlobalValue.vi" "WIFIPW"() -> (w626:string)
                      n263 = To Upper Case(1:w626) -> (0:w623:string)
                      n264 = Match Pattern(string=w625, regular expression=w623) -> (match substring=w624:string)  [unwired: 1 in, 3 out]
                      n265 = Equal?(x=w624, y=w623) -> (x = y?=w630:bool)
                      n266 = Select(t="PASS" ("string"), s=w630, f="FAIL") -> (s? t:f=w627:string)
                    }
                    frame "读出长丰主机条码", "读出五菱主机条码" {
                      n267 = To Upper Case(1:w635) -> (0:w636:string)
                      n268 = String Subset(string=w634, offset (0)=1 ("偏移量(0)")) -> (substring=w632:string)  [unwired: 1 in]
                      n269 = Equal?(x=w632, y=w636) -> (x = y?=w640:bool)
                      n270 = Select(t="PASS" ("string"), s=w640, f="FAIL") -> (s? t:f=w637:string)
                    }
                    frame "读出CCID" {
                      n271 = String Subset(string=w653, offset (0)=1 ("偏移量(0)")) -> (substring=w651:string)  [unwired: 1 in]
                      n272 = To Upper Case(1:w651) -> (0:w642:string)
                      "CCID" <- w642
                      n273 = String Length(string=w642) -> (length=w648:i32)
                      n274 = Equal?(x=w648, y=20) -> (x = y?=w646:bool)
                      n275 = Select(t="PASS" ("string"), s=w646, f="FAIL") -> (s? t:f=w645:string)
                      n276 = call "ccidinfo-w.vi"("Data"=w642, "Data Type"=PDINFO."CCID", "Slot"=w644) -> ()  [unwired: 1 in]
                    }
                    frame "读出生产日期" {
                      n277 = Equal?(x=w660, y=w655) -> (x = y?=w659:bool)
                      n278 = Select(t="PASS" ("string"), s=w659, f="FAIL") -> (s? t:f=w656:string)
                    }
                    frame "读出终端ID" {
                      n279 = String Subset(string=w663, offset (0)=1 ("偏移量(0)")) -> (substring=w662:string)  [unwired: 1 in]
                      n280 = Equal?(x=w662, y=w665) -> (x = y?=w669:bool)
                      n281 = Select(t="PASS" ("string"), s=w669, f="FAIL") -> (s? t:f=w666:string)
                    }
                    frame "读出硬件版本" {
                      n282 = call "Set HW data.vi"("Slot"=w672) -> ("HW DATA"=w671:string)  [unwired: 4 in]
                      n283 = String Subset(string=w674, offset (0)=1 ("偏移量(0)")) -> (substring=w673:string)  [unwired: 1 in]
                      n284 = Equal?(x=w673, y=w671) -> (x = y?=w679:bool)
                      n285 = Select(t="PASS" ("string"), s=w679, f="FAIL") -> (s? t:f=w676:string)
                    }
                  }
                }
              }
              "data" <- w388
              "字符串数值" <- w387
            }
            frame False {
            }
          }
          n286 = VISA Close(VISA resource name=w368, error in (no error)=w369) -> (error out=w366:errorcluster)
        }
        frame #2 {
          n287 = Tick Count (ms)() -> (millisecond timer value=w715:u32)
        }
        frame #3 {
          w737 = "\r\n"
          n288 = local read "命令"() -> (w733:string)
          n289 = local read "响应"() -> (w718:string)
          n290 = String To Byte Array(string=w733) -> (unsigned byte array=w734:u8[])
          n291 = case shown="\"假\", 默认" w717 {
            tunnel: [w742 w750 w751] -> w728
            tunnel: w718 -> [w741 w750 w751]
            frame "假", Default {
              n292 = String To Byte Array(string=w741) -> (unsigned byte array=w744:u8[])
              n293 = for {
                tunnel: w744 -> [w749] mode=indexing
                shift-right: [w747] -> w742
                shift-left: "" -> [w746]
                n294 = Number To Hexadecimal String(1:i16 2 ("宽度(-)"), 2:w749) -> (0:w748:string)
                n295 = Concatenate Strings(w746, w748) -> (w747:string)
              }
            }
            frame "启动自动化测试" {
            }
            frame "查询版本", "查询版本(长丰)" {
            }
          }
          n296 = for {
            tunnel: w734 -> [w760] mode=indexing
            shift-right: [w758] -> w732
            shift-left: "" -> [w757]
            n297 = Number To Hexadecimal String(1:i16 2 ("宽度(-)"), 2:w760) -> (0:w759:string)
            n298 = Concatenate Strings(w757, w759) -> (w758:string)
          }
          n299 = Unbundle By Name(w729) -> ("code"=w724:i32)
          n300 = Equal?(x=w724, y=-1073807253) -> (x = y?=w725:bool)
          n301 = Equal?(x=w724, y=-1073807298) -> (x = y?=w722:bool)
          n302 = Equal?(x=w724, y=-1073807252) -> (x = y?=w719:bool)
          n303 = Or(x=w725, y=w722) -> (x .or. y?=w720:bool)
          n304 = Or(x=w720, y=w719) -> (x .or. y?=w721:bool)
          n305 = case shown="假" w721 {
            tunnel: [w753 errorcluster {"status"=FALSE, "code"=0, "source"=""} ("t")] -> w730
            tunnel: w729 -> [w753 _]
            tunnel: w728 -> [w752 _]
            tunnel: [w752 ""] -> w727
            frame False {
            }
            frame True {
            }
          }
          n306 = Concatenate Strings("发送" ("字符串"), w717, ":" ("字符串"), w732, w737, "反馈:" ("字符串"), w727, w737) -> (→"CMD":string)
        }
        frame #4 {
          n307 = Tick Count (ms)() -> (millisecond timer value=w761:u32)
        }
      }
    }
  }
  "error out" <- w70
  n308 = Subtract(x=w66, y=w48) -> (x-y=→"x-y":u32)
